vi "Interpolate s-parameters.vi"() -> ()   [LabVIEW 2020]
uses:
  <vilib>/Analysis/1siggen.llb/Ramp Pattern by Samples.vi
  <vilib>/addons/HF Network Analysis/Support VIs/Read SnP File (SnP).vi
  <vilib>/Analysis/NI_AALBase.lvlib
  <vilib>/gmath/NI_Gmath.lvlib
  <vilib>/addons/HF Network Analysis/NI_HFNetworkAnalysis.lvlib
panel:
  in  "samples":i32=3999
  out "error":i32
  in  "S1P File Path":path
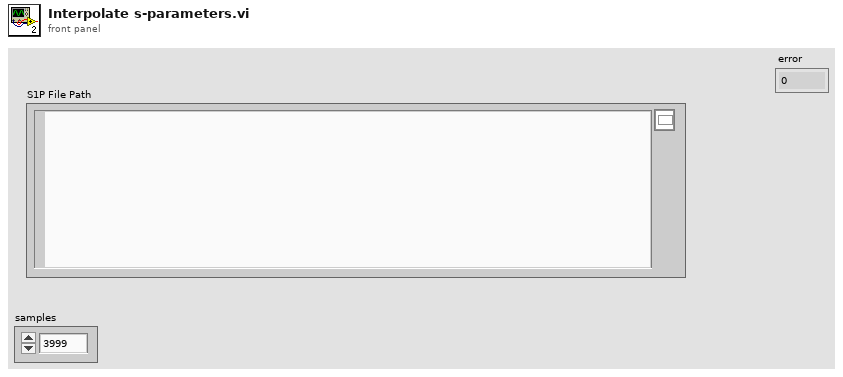
[diagram p1: front panel]
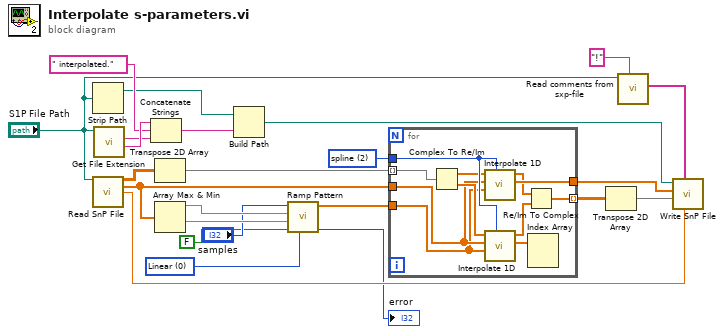
[diagram p0: block diagram]
diagram:
  w3 = u16 0 items=["Linear", "Logarithmic"] ("type")
  w21 = 2 items=["nearest", "linear", "spline", "cubic Hermite", "Lagrange"] ("method")
  n1 = Strip Path(path="S1P File Path") -> (stripped path=w13:path)  [unwired: 1 out]
  n2 = call-poly <vilib>:"Read SnP File.vi"("SnP File Path"="S1P File Path") -> ("S-parameters"=w7:cdb[][], "Frequencies (Hz)"=w20:dbl[], "Z0 (Ohm)"=w8:cdb)  [unwired: 11 in, 1 out]
  n3 = call <vilib>:"Get File Extension.vi"("file"="S1P File Path") -> ("filename without extension"=w17:string, "lowercase file extension"=w15:string)  [unwired: 6 in, 3 out]
  n4 = Concatenate Strings(w17, " interpolated." ("string"), w15) -> (w14:string)
  n5 = Transpose 2D Array(2D array=w7) -> (transposed array=w6:cdb[][])
  n6 = Array Max & Min(array=w20) -> (max value=w23:dbl, min value=w24:dbl)  [unwired: 2 out]
  n7 = Build Path(base path=w13, name or relative path=w14) -> (appended path=w12:path)
  n8 = call-poly <vilib>:"Ramp Pattern.vi"("type"=w3, "exclude end?"=FALSE, "start"=w24, "end"=w23, "samples"="samples") -> ("error"=→"error":i32, "Ramp Pattern"=w19:dbl[])  [unwired: 5 in]
  n9 = for {
    tunnel: w21 -> [w34]
    tunnel: w6 -> [w31] mode=indexing
    tunnel: w20 -> [w30]
    tunnel: w19 -> [w29]
    tunnel: [w28] -> w18
    tunnel: [w25] -> w5 mode=indexing
    n10 = Complex To Re/Im(x + iy=w31) -> (x=w33:dbl[], y=w32:dbl[])
    n11 = call <vilib>:"Interpolate 1D.vi"("method"=w34, "xi"=w29, "X"=w30, "Y"=w33) -> ("xi used"=w28:dbl[], "yi"=w26:dbl[])  [unwired: 5 in, 1 out]
    n12 = call <vilib>:"Interpolate 1D.vi"("method"=w34, "xi"=w29, "X"=w30, "Y"=w32) -> ("xi used"=w35:dbl[], "yi"=w27:dbl[])  [unwired: 5 in, 1 out]
    n13 = Re/Im To Complex(1:w27, 2:w26) -> (0:w25:cdb[])
    n14 = Index Array(array=w35) -> ()  [unwired: 2 in, 2 out]
  }
  n15 = Transpose 2D Array(2D array=w5) -> (transposed array=w4:cdb[][])
  n16 = call "Read comments from sxp-file.vi"("Comment character"="!", "file path"="S1P File Path") -> ("Comment lines"=w9:string[])  [unwired: 7 in, 2 out]
  n17 = call <vilib>:"Write SnP File.vi"("Z0 (50 Ohm)"=w8, "Comments"=w9, "S-parameters"=w4, "Frequencies (Hz)"=w18, "SnP File Path"=w12) -> ()  [unwired: 6 in, 1 out]
